vi "DisplayExecution Event Callback.vi"(4 "cluster":T1, 5 "Event data":cluster{"exec":refnum<k7>, "reason":i32}, 6 "CtlRef":refnum<k7>, 7 "Event common data":cluster{"Source":i32, "Type":u32, "Time":u32}) -> ()   [LabVIEW 2025]
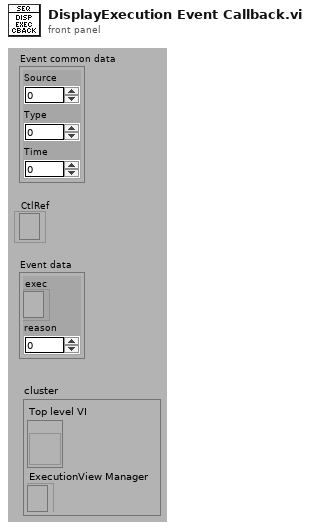
[diagram p1: front panel]
types:
  T1 = cluster{"Top level VI":refnum<vi>, "ExecutionView Manager":refnum<k7>}
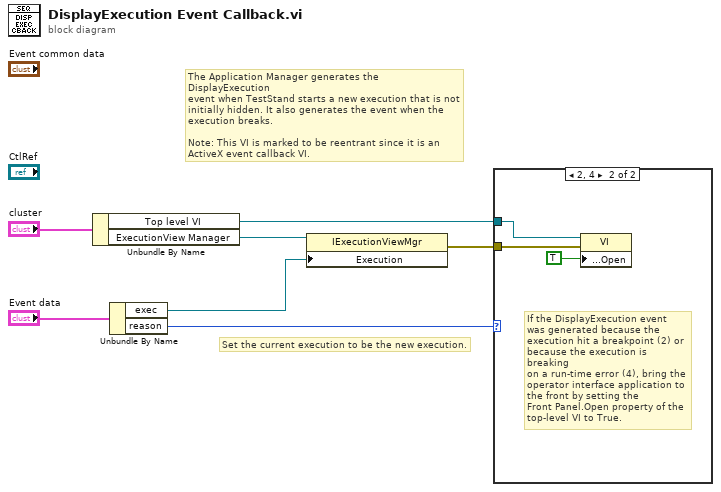
[diagram p0: block diagram]
diagram:
  # "The Application Manager generates the DisplayExecution\nevent when TestStand starts a new execution that is not\ninitially hidden. It also generates the event when the\nexecution breaks.\n\nNote: This VI is marked to be reentrant since it is an\nActiveX event callback VI."
  # "Set the current execution to be the new execution."
  n1 = Unbundle By Name("cluster") -> ("Top level VI"=w4:refnum<vi>, "ExecutionView Manager"=w3:refnum<k7>)
  n2 = Unbundle By Name("Event data") -> ("exec"=w7:refnum<k7>, "reason"=w1:i32)
  n3 = property class="IExecutionViewMgr"(reference=w3, "Execution"=w7) -> (error out=w5:errorcluster)  [unwired: 1 in, 1 out]
  n4 = case shown="2, 4" w1 {
    tunnel: w5 -> [_ w10]
    tunnel: w4 -> [_ w8]
    frame Default {
    }
    frame 2, 4 {
      # "If the DisplayExecution event\nwas generated because the\nexecution hit a breakpoint (2) or\nbecause the execution is breaking\non a run-time error (4), bring the\noperator interface application to\nthe front by setting the\nFront Panel.Open property of the\ntop-level VI to True."
      n5 = property class="VI"(reference=w8, error in=w10, "Front Panel Window:Open"=TRUE) -> ()  [unwired: 2 out]
    }
  }
